vi "easing_CubicIn.vi"(9 "distance":dbl, 10 "interval (10 ms)":dbl, 11 "time":dbl) -> (3 "current position":dbl)   [LabVIEW 2023]
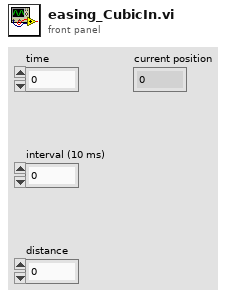
[diagram p1: front panel]
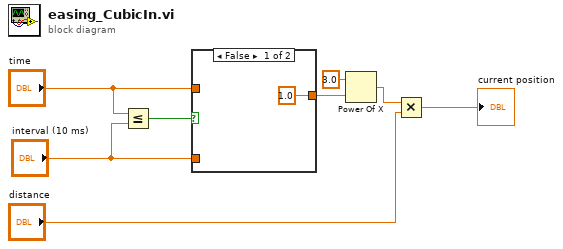
[diagram p0: block diagram]
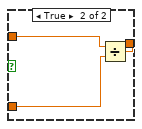
[diagram p2: hidden frame]
diagram:
  n1 = Less Or Equal?(x="time", y="interval (10 ms)") -> (x <= y?=w1:bool)
  n2 = case shown="False" w1 {
    tunnel: [1.0 ("y") w12] -> w5
    tunnel: "interval (10 ms)" -> [_ w11]
    tunnel: "time" -> [_ w10]
    frame False {
    }
    frame True {
      n3 = Divide(x=w10, y=w11) -> (x/y=w12:dbl)
    }
  }
  n4 = Power Of X(1:w5, 2:3.0 ("y")) -> (0:w6:dbl)
  n5 = Multiply(x=w6, y="distance") -> (x*y=→"current position":dbl)
